vi "Core.vi"(10 "Class Return Notifier":refnum<notifier>, 11 "Engine in":refnum<class "Engine.lvclass">) -> ()   [LabVIEW 2020, in "GLF.lvlib" / "Engine.lvclass"]
doc: "<B>Summary</B>\nThe GLF main process handling SDL events and clients commands."
uses:
  Engine.lvclass
  Engine.lvclass/Engine.ctl
  <vilib>/Saukko/LV SDL3/Sources/SDL3/Timer/Timer.lvlib
  IAmGLF/IAmGLF.lvclass
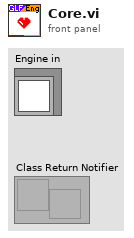
[diagram p1: front panel]
types:
  T1 = typedef "GLF.lvlib/Engine.lvclass/DVR--cluster.ctl" = cluster{"CMD Queue":T2, "Config":T3, "Ctxt":T5, "Metrics":T6, "Debug":T7, "ID To Window":map{T9, refnum<class "Window.lvclass">}, "Window To Handle":map{refnum<class "Window.lvclass">, i64}}
  T2 = typedef "GLF.lvlib/Engine.lvclass/Command--queue.ctl" = refnum<queue>
  T3 = typedef "GLF.lvlib/Engine.lvclass/Config--cluster.ctl" = cluster{"Quit On Last Window Closed":bool, "VSync":T4, "FPS Target":dbl}
  T4 = typedef "GLF.lvlib/Engine.lvclass/VSync--enum.ctl" = enum16{"Disabled", "Enabled", "Adaptative"}
  T5 = typedef "GLF.lvlib/Engine.lvclass/Context--cluster.ctl" = cluster{"VSync Enabled":bool}
  T6 = typedef "GLF.lvlib/Engine.lvclass/Metrics--cluster.ctl" = cluster{"Uptime [ms]":u64, "Loop Time [ms]":u64, "Timer [ns]":u64, "Poll Events [ns]":u64, "Dequeue CMD [ns]":u64, "Update Layout [ns]":u64, "Render [ns]":u64}
  T7 = typedef "GLF.lvlib/Engine.lvclass/Debug--cluster.ctl" = cluster{"Unhandled Events":map{T8, u64}}
  T8 = typedef "SDL3.lvlib/Events.lvlib/EventType--enum.ctl" = enum16{"LV_NONE", "LV_UNSUPPORTED", "SDL_EVENT_QUIT", "SDL_EVENT_LOCALE_CHANGED", "SDL_EVENT_SYSTEM_THEME_CHANGED", "SDL_EVENT_DISPLAY_ORIENTATION", "SDL_EVENT_DISPLAY_ADDED", "SDL_EVENT_DISPLAY_REMOVED", "SDL_EVENT_DISPLAY_MOVED", "SDL_EVENT_DISPLAY_DESKTOP_MODE_CHANGED", "SDL_EVENT_DISPLAY_CURRENT_MODE_CHANGED", "SDL_EVENT_DISPLAY_CONTENT_SCALE_CHANGED", "SDL_EVENT_WINDOW_SHOWN", "SDL_EVENT_WINDOW_HIDDEN", "SDL_EVENT_WINDOW_EXPOSED", "SDL_EVENT_WINDOW_MOVED", "SDL_EVENT_WINDOW_RESIZED", "SDL_EVENT_WINDOW_PIXEL_SIZE_CHANGED", "SDL_EVENT_WINDOW_METAL_VIEW_RESIZED", "SDL_EVENT_WINDOW_MINIMIZED", "SDL_EVENT_WINDOW_MAXIMIZED", "SDL_EVENT_WINDOW_RESTORED", "SDL_EVENT_WINDOW_MOUSE_ENTER", "SDL_EVENT_WINDOW_MOUSE_LEAVE", "SDL_EVENT_WINDOW_FOCUS_GAINED", "SDL_EVENT_WINDOW_FOCUS_LOST", "SDL_EVENT_WINDOW_CLOSE_REQUESTED", "SDL_EVENT_WINDOW_HIT_TEST", "SDL_EVENT_WINDOW_ICCPROF_CHANGED", "SDL_EVENT_WINDOW_DISPLAY_CHANGED", "SDL_EVENT_WINDOW_DISPLAY_SCALE_CHANGED", "SDL_EVENT_WINDOW_SAFE_AREA_CHANGED", "SDL_EVENT_WINDOW_OCCLUDED", "SDL_EVENT_WINDOW_ENTER_FULLSCREEN", "SDL_EVENT_WINDOW_LEAVE_FULLSCREEN", "SDL_EVENT_WINDOW_DESTROYED", "SDL_EVENT_WINDOW_HDR_STATE_CHANGED", "SDL_EVENT_KEY_DOWN", "SDL_EVENT_KEY_UP", "SDL_EVENT_TEXT_EDITING", "SDL_EVENT_TEXT_INPUT", "SDL_EVENT_KEYMAP_CHANGED", "SDL_EVENT_KEYBOARD_ADDED", "SDL_EVENT_KEYBOARD_REMOVED", "SDL_EVENT_TEXT_EDITING_CANDIDATES", "SDL_EVENT_MOUSE_MOTION", "SDL_EVENT_MOUSE_BUTTON_DOWN", "SDL_EVENT_MOUSE_BUTTON_UP", "SDL_EVENT_MOUSE_WHEEL", "SDL_EVENT_MOUSE_ADDED", "SDL_EVENT_MOUSE_REMOVED", "SDL_EVENT_JOYSTICK_AXIS_MOTION", "SDL_EVENT_JOYSTICK_BALL_MOTION", "SDL_EVENT_JOYSTICK_HAT_MOTION", "SDL_EVENT_JOYSTICK_BUTTON_DOWN", "SDL_EVENT_JOYSTICK_BUTTON_UP", "SDL_EVENT_JOYSTICK_ADDED", "SDL_EVENT_JOYSTICK_REMOVED", "SDL_EVENT_JOYSTICK_BATTERY_UPDATED", "SDL_EVENT_JOYSTICK_UPDATE_COMPLETE", "SDL_EVENT_GAMEPAD_AXIS_MOTION", "SDL_EVENT_GAMEPAD_BUTTON_DOWN", "SDL_EVENT_GAMEPAD_BUTTON_UP", "SDL_EVENT_GAMEPAD_ADDED", "SDL_EVENT_GAMEPAD_REMOVED", "SDL_EVENT_GAMEPAD_REMAPPED", "SDL_EVENT_GAMEPAD_TOUCHPAD_DOWN", "SDL_EVENT_GAMEPAD_TOUCHPAD_MOTION", "SDL_EVENT_GAMEPAD_TOUCHPAD_UP", "SDL_EVENT_GAMEPAD_SENSOR_UPDATE", "SDL_EVENT_GAMEPAD_UPDATE_COMPLETE", "SDL_EVENT_GAMEPAD_STEAM_HANDLE_UPDATED", "SDL_EVENT_FINGER_DOWN", "SDL_EVENT_FINGER_UP", "SDL_EVENT_FINGER_MOTION", "SDL_EVENT_CLIPBOARD_UPDATE", "SDL_EVENT_DROP_FILE", "SDL_EVENT_DROP_TEXT", "SDL_EVENT_DROP_BEGIN", "SDL_EVENT_DROP_COMPLETE", "SDL_EVENT_DROP_POSITION", "SDL_EVENT_AUDIO_DEVICE_ADDED", "SDL_EVENT_AUDIO_DEVICE_REMOVED", "SDL_EVENT_AUDIO_DEVICE_FORMAT_CHANGED", "SDL_EVENT_SENSOR_UPDATE", "SDL_EVENT_PEN_PROXIMITY_IN", "SDL_EVENT_PEN_PROXIMITY_OUT", "SDL_EVENT_PEN_DOWN", "SDL_EVENT_PEN_UP", "SDL_EVENT_PEN_BUTTON_DOWN", "SDL_EVENT_PEN_BUTTON_UP", "SDL_EVENT_PEN_MOTION", "SDL_EVENT_PEN_AXIS", "SDL_EVENT_CAMERA_DEVICE_ADDED", "SDL_EVENT_CAMERA_DEVICE_REMOVED", "SDL_EVENT_CAMERA_DEVICE_APPROVED", "SDL_EVENT_CAMERA_DEVICE_DENIED", "SDL_EVENT_RENDER_TARGETS_RESET", "SDL_EVENT_RENDER_DEVICE_RESET", "SDL_EVENT_POLL_SENTINEL", "SDL_EVENT_USER"}
  T9 = typedef "SDL3.lvlib/Video.lvlib/WindowID--integer.ctl" = u32
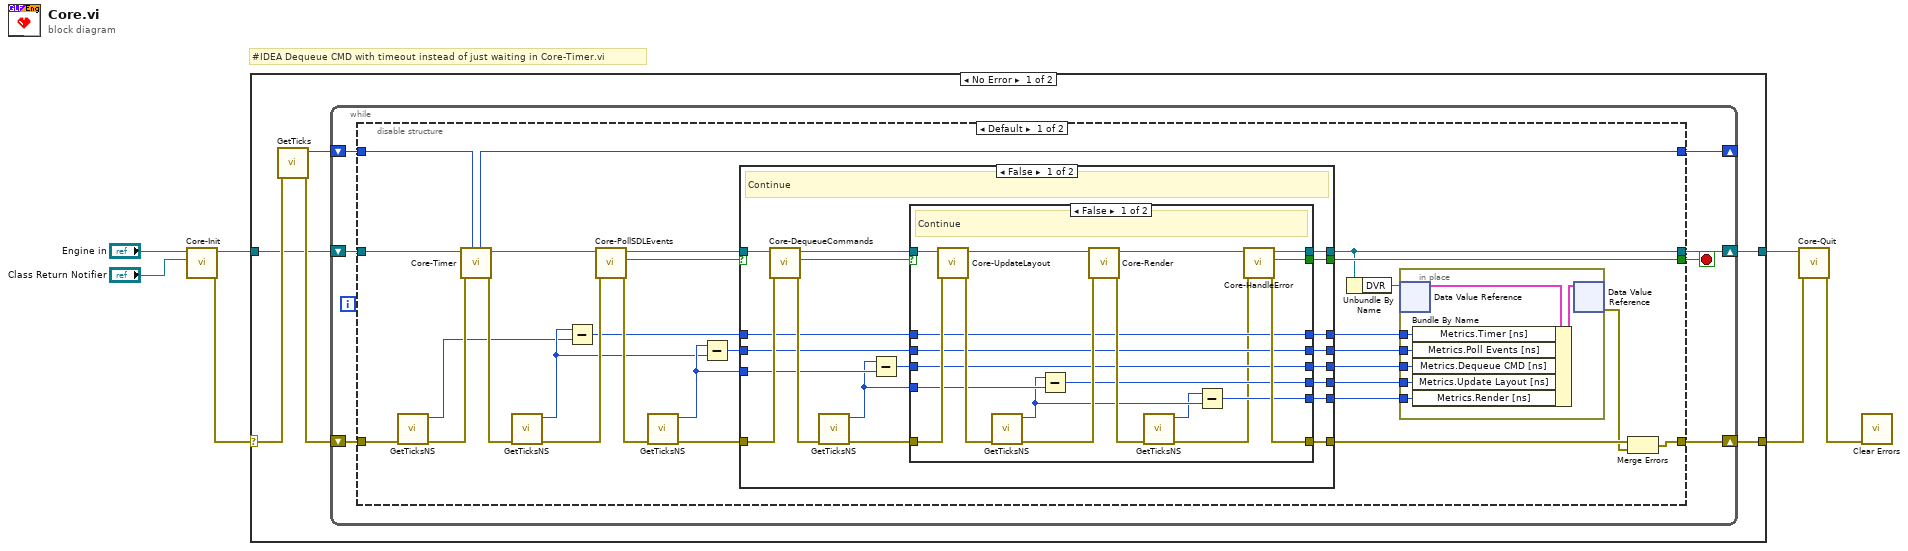
[diagram p0: block diagram]
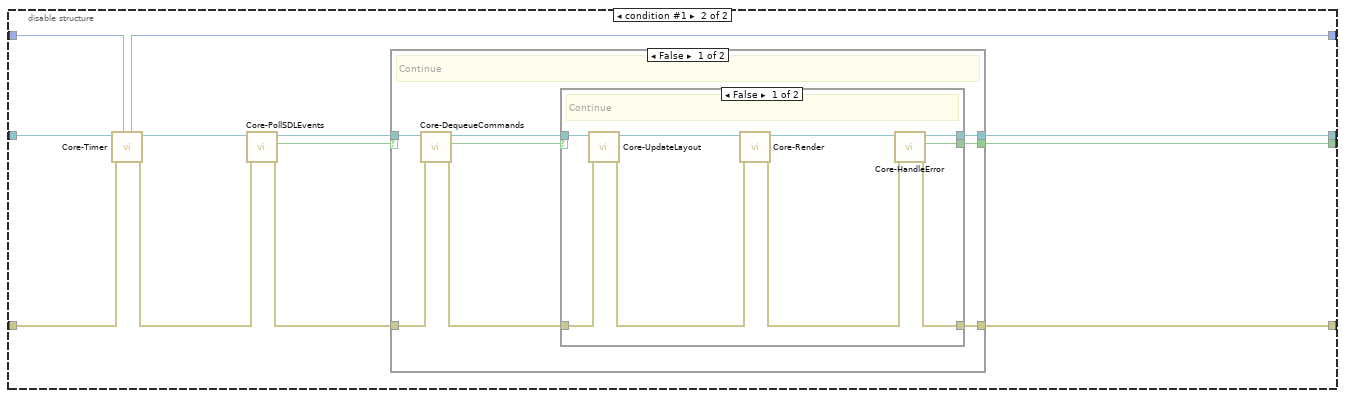
[diagram p4: hidden frame]
diagram:
  # "#IDEA Dequeue CMD with timeout instead of just waiting in Core-Timer.vi"
  n1 = call "Core-Init.vi"("Class Return Notifier"="Class Return Notifier", "Engine in"="Engine in") -> ("error out"=w5:errorcluster, "Engine out"=w6:refnum<class "Engine.lvclass">)  [unwired: 8 in]
  n2 = case shown="No Error" w5 {
    selector: w5 -> [w13 w141]
    tunnel: w6 -> [w11 w140]
    tunnel: [w10 w140] -> w4
    tunnel: [w9 w141] -> w3
    frame No Error {
      n3 = call <vilib>:"GetTicks.vi"("No Error"=w13) -> ("error out"=w12:errorcluster, "Ticks [ms]"=w8:u64)  [unwired: 9 in]
      n4 = while {
        shift-right: [w17] -> w10
        shift-left: w11 -> [w20]
        shift-right: [w16] -> w9
        shift-left: w12 -> [w19]
        shift-right: [w14] -> _
        shift-left: w8 -> [w15]
        stop <- w18 stop-if-true
        n5 = disable-structure shown="Default" {
          disable-tunnel: w20 -> [w48 w116]
          disable-tunnel: w19 -> [w43 w107]
          disable-tunnel: [w41 w113] -> w18
          disable-tunnel: [w35 w111] -> w17
          disable-tunnel: [w29 w108] -> w16
          disable-tunnel: w15 -> [w22 w110]
          disable-tunnel: [w21 w109] -> w14
          frame condition #0 (active) {
            n6 = call <vilib>:"GetTicksNS.vi"("No Error"=w43) -> ("error out"=w27:errorcluster, "Ticks [ns]"=w25:u64)  [unwired: 9 in]
            n7 = call "Core-Timer.vi"("Ticks Begin In [ms]"=w22, "error in (no error)"=w27, "Engine in"=w48) -> ("error out"=w42:errorcluster, "Engine out"=w44:refnum<class "Engine.lvclass">, "Ticks Begin Out [ms]"=w21:u64)  [unwired: 6 in]
            n8 = call <vilib>:"GetTicksNS.vi"("No Error"=w42) -> ("error out"=w40:errorcluster, "Ticks [ns]"=w26:u64)  [unwired: 9 in]
            n9 = Subtract(x=w26, y=w25) -> (x-y=w23:u64)
            n10 = call "Core-PollSDLEvents.vi"("error in (no error)"=w40, "Engine in"=w44) -> ("error out"=w46:errorcluster, "Quit?"=w38:bool, "Engine out"=w47:refnum<class "Engine.lvclass">)  [unwired: 7 in]
            n11 = call <vilib>:"GetTicksNS.vi"("No Error"=w46) -> ("error out"=w39:errorcluster, "Ticks [ns]"=w37:u64)  [unwired: 9 in]
            n12 = Subtract(x=w37, y=w26) -> (x-y=w36:u64)
            n13 = case shown="False" w38 {
              selector: w38 -> [_ w97]
              tunnel: w47 -> [w67 w96]
              tunnel: [w65 w96] -> w35
              tunnel: [w63 w94] -> w45
              tunnel: [w61 w97] -> w41
              tunnel: w39 -> [w60 w94]
              tunnel: w37 -> [w57 _]
              tunnel: w36 -> [w58 w95]
              tunnel: [w54 w95] -> w33
              tunnel: [w53 _] -> w32
              tunnel: [w52 _] -> w31
              tunnel: [w51 _] -> w30
              tunnel: [w50 w93] -> w24
              tunnel: w23 -> [w49 w93]
              frame False {
                # "Continue"
                n14 = call "Core-DequeueCommands.vi"("error in (no error)"=w60, "Engine in"=w67) -> ("error out"=w64:errorcluster, "Quit?"=w62:bool, "Engine out"=w66:refnum<class "Engine.lvclass">)  [unwired: 7 in]
                n15 = call <vilib>:"GetTicksNS.vi"("No Error"=w64) -> ("error out"=w59:errorcluster, "Ticks [ns]"=w56:u64)  [unwired: 9 in]
                n16 = Subtract(x=w56, y=w57) -> (x-y=w55:u64)
                n17 = case shown="False" w62 {
                  selector: w62 -> [_ w90]
                  tunnel: w66 -> [w86 w92]
                  tunnel: [w82 w92] -> w65
                  tunnel: w59 -> [w78 w91]
                  tunnel: [w81 w91] -> w63
                  tunnel: [w80 w90] -> w61
                  tunnel: w56 -> [w75 _]
                  tunnel: w58 -> [w77 w89]
                  tunnel: [w77 w89] -> w54
                  tunnel: w55 -> [w76 w88]
                  tunnel: [w76 w88] -> w53
                  tunnel: [w74 _] -> w52
                  tunnel: [w71 _] -> w51
                  tunnel: [w70 w87] -> w50
                  tunnel: w49 -> [w70 w87]
                  frame False {
                    # "Continue"
                    n18 = call "Core-UpdateLayout.vi"("error in (no error)"=w78, "Engine in"=w86) -> ("error out"=w83:errorcluster, "Engine out"=w84:refnum<class "Engine.lvclass">)  [unwired: 8 in]
                    n19 = call <vilib>:"GetTicksNS.vi"("No Error"=w83) -> ("error out"=w79:errorcluster, "Ticks [ns]"=w73:u64)  [unwired: 9 in]
                    n20 = Subtract(x=w73, y=w75) -> (x-y=w74:u64)
                    n21 = call "Core-Render.vi"("error in (no error)"=w79, "Engine in"=w84) -> ("error out"=w85:errorcluster, "Engine out"=w69:refnum<class "Engine.lvclass">)  [unwired: 8 in]
                    n22 = call <vilib>:"GetTicksNS.vi"("No Error"=w85) -> ("error out"=w68:errorcluster, "Ticks [ns]"=w72:u64)  [unwired: 9 in]
                    n23 = Subtract(x=w72, y=w73) -> (x-y=w71:u64)
                    n24 = call "Core-HandleError.vi"("error in (no error)"=w68, "Engine in"=w69) -> ("error out"=w81:errorcluster, "Quit?"=w80:bool, "Engine out"=w82:refnum<class "Engine.lvclass">)  [unwired: 7 in]
                  }
                  frame True {
                    # "Quit"
                  }
                }
              }
              frame True {
                # "Quit"
              }
            }
            n25 = Unbundle By Name(w35) -> ("DVR"=w34:refnum<data-value>)
            n26 = in-place {
              in-place-border: w33 -> [w102]
              in-place-border: w32 -> [w101]
              in-place-border: w31 -> [w100]
              in-place-border: w30 -> [w99]
              in-place-border: w24 -> [w98]
              n27 = in-place-dvr #1(w34) -> (w104:T1)  [unwired: 1 out]
              n28 = Bundle By Name(cluster=w104, "Metrics.Timer [ns]"=w98, "Metrics.Poll Events [ns]"=w102, "Metrics.Dequeue CMD [ns]"=w101, "Metrics.Update Layout [ns]"=w100, "Metrics.Render [ns]"=w99) -> (w103:T1)
              n29 = in-place-dvr #1(w103) -> (w28:errorcluster)  [unwired: 1 out]
            }
            n30 = Merge Errors(w45, w28) -> (w29:errorcluster)
          }
          frame condition #1 {
            n31 = call "Core-Timer.vi"("Ticks Begin In [ms]"=w110, "error in (no error)"=w107, "Engine in"=w116) -> ("error out"=w106:errorcluster, "Engine out"=w114:refnum<class "Engine.lvclass">, "Ticks Begin Out [ms]"=w109:u64)  [unwired: 6 in]
            n32 = call "Core-PollSDLEvents.vi"("error in (no error)"=w106, "Engine in"=w114) -> ("error out"=w105:errorcluster, "Quit?"=w112:bool, "Engine out"=w115:refnum<class "Engine.lvclass">)  [unwired: 7 in]
            n33 = case shown="False" w112 {
              selector: w112 -> [_ w139]
              tunnel: w115 -> [w124 w138]
              tunnel: [w122 w138] -> w111
              tunnel: [w121 w137] -> w108
              tunnel: [w119 w139] -> w113
              tunnel: w105 -> [w118 w137]
              frame False {
                # "Continue"
                n34 = call "Core-DequeueCommands.vi"("error in (no error)"=w118, "Engine in"=w124) -> ("error out"=w117:errorcluster, "Quit?"=w120:bool, "Engine out"=w123:refnum<class "Engine.lvclass">)  [unwired: 7 in]
                n35 = case shown="False" w120 {
                  selector: w120 -> [_ w134]
                  tunnel: w123 -> [w133 w136]
                  tunnel: [w131 w136] -> w122
                  tunnel: w117 -> [w128 w135]
                  tunnel: [w130 w135] -> w121
                  tunnel: [w129 w134] -> w119
                  frame False {
                    # "Continue"
                    n36 = call "Core-UpdateLayout.vi"("error in (no error)"=w128, "Engine in"=w133) -> ("error out"=w126:errorcluster, "Engine out"=w132:refnum<class "Engine.lvclass">)  [unwired: 8 in]
                    n37 = call "Core-Render.vi"("error in (no error)"=w126, "Engine in"=w132) -> ("error out"=w125:errorcluster, "Engine out"=w127:refnum<class "Engine.lvclass">)  [unwired: 8 in]
                    n38 = call "Core-HandleError.vi"("error in (no error)"=w125, "Engine in"=w127) -> ("error out"=w130:errorcluster, "Quit?"=w129:bool, "Engine out"=w131:refnum<class "Engine.lvclass">)  [unwired: 7 in]
                  }
                  frame True {
                    # "Quit"
                  }
                }
              }
              frame True {
                # "Quit"
              }
            }
          }
        }
      }
    }
    frame Error {
    }
  }
  n39 = call "Core-Quit.vi"("error in (no error)"=w3, "Engine in"=w4) -> ("error out"=w2:errorcluster)  [unwired: 9 in]
  n40 = call <vilib>:"Clear Errors.vi"("error in (no error)"=w2) -> ()  [unwired: 5 in, 2 out]
